vi "Save Macro.vi"(8 "error in (no error)":errorcluster, 10 "Macro Cluster":T1, 11 "File Path":path) -> (0 "error out":errorcluster)   [LabVIEW 2020, in "MacroAssert.lvlib"]
doc: "Saves <B>Macro Cluster</B> and its associated <B>Macro Name</B> to an INI file located in <B>App Data Directory</B>."
uses:
  MacroAssert.lvlib
  CTLs/Macro Cluster V3.ctl
  CTLs/Macro Config V3.ctl
  CTLs/Step V3.ctl
  CTLs/Step Type V3.ctl
  <vilib>/Utility/config.llb/NI_LVConfig.lvlib
  <userlib>/_OpenG.lib/file/file.llb/openg_file.lvlib
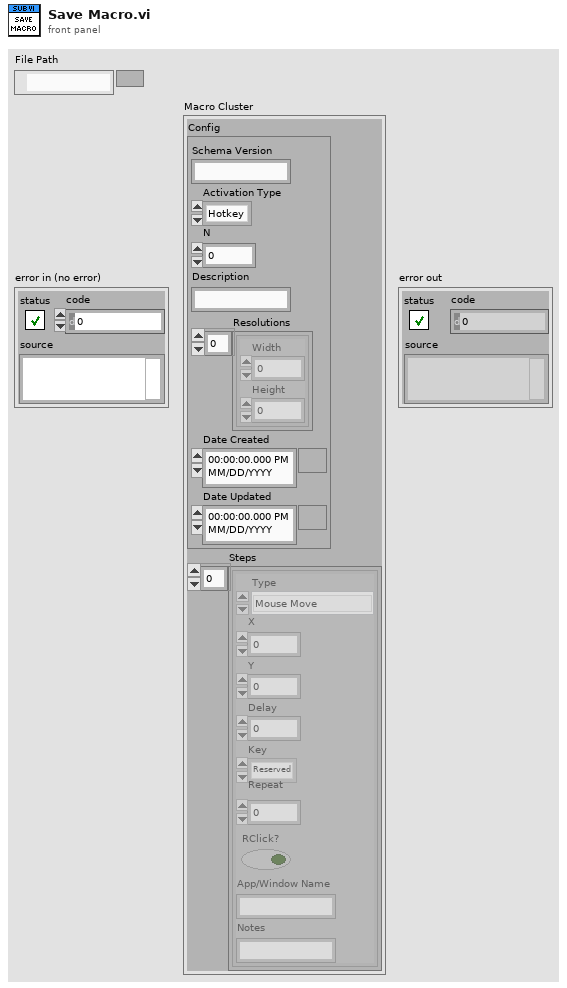
[diagram p1: front panel]
types:
  T1 = typedef "MacroAssert.lvlib/Macro Cluster V3.ctl" = cluster{"Config":T2, "Steps":T3[]}
  T2 = typedef "MacroAssert.lvlib/Macro Config V3.ctl" = cluster{"Schema Version":string, "Activation Type":enum32{"Hotkey", "Automatic"}, "N":i32, "Description":string, "Resolutions":cluster{"Width":i16, "Height":i16}[], "Date Created":timestamp, "Date Updated":timestamp}
  T3 = typedef "MacroAssert.lvlib/Step V3.ctl" = cluster{"Type":T4, "X":i32, "Y":i32, "Delay":i32, "Key":u8, "Repeat":i32, "RClick?":bool, "App/Window Name":string, "Notes":string}
  T4 = typedef "MacroAssert.lvlib/Step Type V3.ctl" = enum16{"Mouse Move", "Mouse Click", "Key Press", "Wait", "Mouse Down", "Mouse Up", "Key Down", "Key Up", "Run Application", "Maximize Window", "Restore Window", "Minimize Window", "Close Window", "Bring Window to Front", "Send Window to Back"}
  T5 = typedef "NI_LVConfig.lvlib/Config Data RefNum.ctl" = refnum<k1>
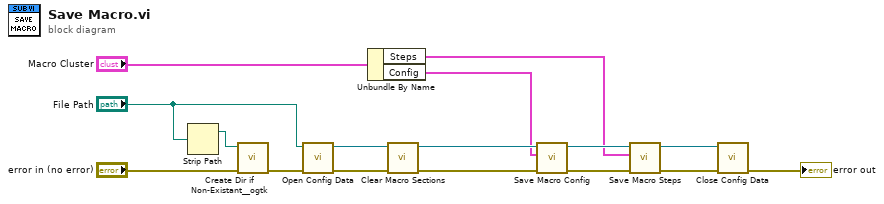
[diagram p0: block diagram]
diagram:
  n1 = Strip Path(path="File Path") -> (stripped path=w2:path)  [unwired: 1 out]
  n2 = call <userlib>:"Create Dir if Non-Existant__ogtk.vi"("error in (no error)"="error in (no error)", "Directory Path"=w2) -> ("error out"=w4:errorcluster)  [unwired: 7 in, 2 out]
  n3 = call <vilib>:"Open Config Data.vi"("error in (no error)"=w4, "configuration file path"="File Path") -> ("error out"=w14:errorcluster, "refnum"=w13:T5)  [unwired: 7 in, 1 out]
  n4 = Unbundle By Name("Macro Cluster") -> ("Steps"=w7:T3[], "Config"=w3:T2)
  n5 = call "Clear Macro Sections.vi"("error in (no error)"=w14, "refnum"=w13) -> ("error out"=w12:errorcluster, "refnum out"=w11:T5)  [unwired: 8 in]
  n6 = call "Save Macro Config.vi"("error in (no error)"=w12, "Macro Config"=w3, "refnum"=w11) -> ("error out"=w9:errorcluster, "refnum out"=w10:T5)  [unwired: 7 in]
  n7 = call "Save Macro Steps.vi"("error in (no error)"=w9, "Macro Steps"=w7, "refnum"=w10) -> ("error out"=w5:errorcluster, "refnum out"=w6:T5)  [unwired: 7 in]
  n8 = call <vilib>:"Close Config Data.vi"("error in (no error)"=w5, "refnum"=w6) -> ("error out"=→"error out":errorcluster)  [unwired: 8 in, 1 out]
